vi "Get Audio File Info (Path).vi"(8 "error in (no error)":errorcluster, 11 "Path In":path) -> (0 "error out":errorcluster, 1 "Audio File Info":T2, 2 "PCM Frame Length":u64, 3 "Path Out":path, 4 "Codec":T1)   [LabVIEW 2020, in "G-Audio.lvlib"]
doc: "Retrieve audio file information. Some codecs (mp3) require the entire file be parsed to accurately determine the length, which can take time for very large files.\n\nSupported codecs: flac, mp3, ogg (vorbis), and wav."
uses:
  G-Audio.lvlib
  Controls/Audio File Info.ctl
  Controls/Audio File Codec.ctl
  Private/Result To Error.vi
  <vilib>/Utility/error.llb/Error Cluster From Error Code.vi
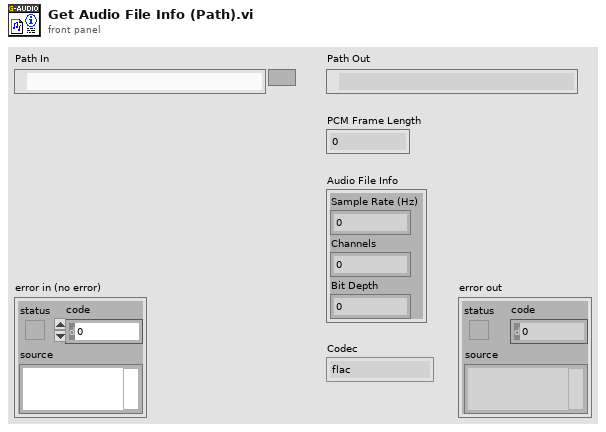
[diagram p1: front panel]
types:
  T1 = typedef "G-Audio.lvlib/Audio File Codec.ctl" = enum16{"flac", "mp3", "vorbis", "wav", "unsupported"}
  T2 = typedef "G-Audio.lvlib/Audio File Info.ctl" = cluster{"Sample Rate (Hz)":u32, "Channels":u32, "Bit Depth":u32}
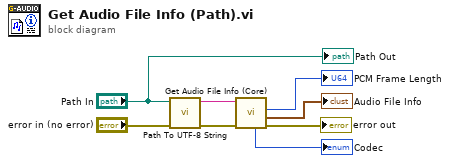
[diagram p0: block diagram]
diagram:
  n1 = call "Path To UTF-8 String.vi"("error in"="error in (no error)", "Path"="Path In") -> ("error out"=w1:errorcluster, "UTF-8 String"=w7:string)  [unwired: 8 in]
  n2 = call "Get Audio File Info (Core).vi"("error in (no error)"=w1, "Path In"=w7) -> ("error out"=→"error out":errorcluster, "Audio File Info"=→"Audio File Info":T2, "PCM Frame Length"=→"PCM Frame Length":u64, "Codec"=→"Codec":T1)  [unwired: 5 in, 1 out]
  "Path Out" <- "Path In"
